vi "Live.Load OPC Tree.vi"(8 "error in (no error)":errorcluster, 9 "Connection.Properties":T1={"Server IP Address"="localhost", "Server Port"=49350, "Message Mode"=enum."None", "Security"=enum."Basic256", "User Name"="", "Password"="", "Client Certificate"=path "", "Server Certificate"=path ""}, 10 "Tree":refnum<vi>, 11 "VI in":refnum<vi>) -> (0 "error out":errorcluster, 3 "LUT":variant)   [LabVIEW 2013, in "OPC UA Client System Explorer.lvlib"]
uses:
  OPC UA Client System Explorer.lvlib
  Shared/Connection.Properties.ctl
  <vilib>/OPCUA/NI OPC UA Client.lvlib
  Shared/OPC UA Client Shared.lvlib
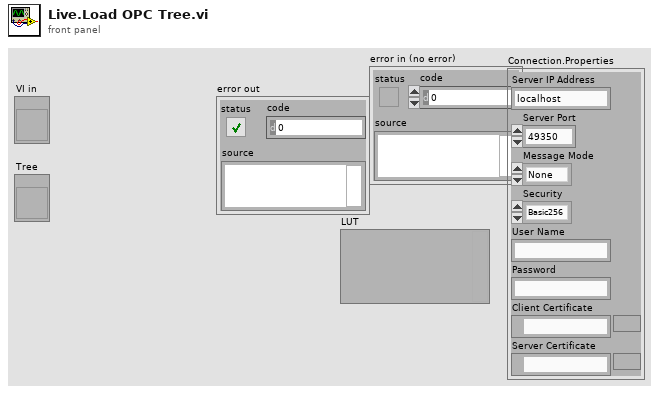
[diagram p1: front panel]
types:
  T1 = typedef "OPC UA Client Shared.lvlib/Connection.Properties.ctl" = cluster{"Server IP Address":string, "Server Port":u16, "Message Mode":enum16{"None", "Sign", "Sign and Encrypt"}, "Security":enum16{"Basic256", "Basic128Rsa15"}, "User Name":string, "Password":string, "Client Certificate":path, "Server Certificate":path}
  T2 = cluster{"message mode":enum16{"None", "Sign", "Sign and Encrypt"}, "security":enum16{"Basic256", "Basic128Rsa15"}}
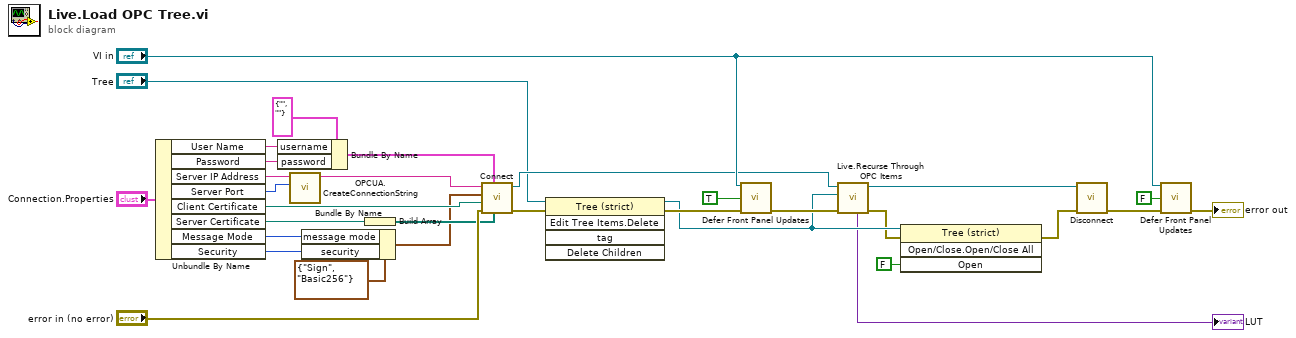
[diagram p0: block diagram]
diagram:
  n1 = Unbundle By Name("Connection.Properties") -> ("User Name"=w11:string, "Password"=w12:string, "Server IP Address"=w15:string, "Server Port"=w14:u16, "Client Certificate"=w8:path, "Server Certificate"=w7:path, "Message Mode"=w3:enum16{"None", "Sign", "Sign and Encrypt"}, "Security"=w2:enum16{"Basic256", "Basic128Rsa15"})
  n2 = Bundle By Name(cluster=cluster{"username":string, "password":string} {"username"="", "password"=""} ("username/password"), "username"=w11, "password"=w12) -> (w9:cluster{"username":string, "password":string})
  n3 = call "OPCUA.CreateConnectionString.vi"("Server Port"=w14, "Server IP Address"=w15) -> ("concatenated string"=w13:string)  [unwired: 9 in]
  n4 = Bundle By Name(cluster=T2 {"message mode"=enum."Sign", "security"=enum."Basic256"} ("security policy"), "message mode"=w3, "security"=w2) -> (w4:T2)
  n5 = Build Array(w7) -> (w6:path[])
  n6 = call <vilib>:"Connect.vi"("trusted server certificates"=w6, "username/password"=w9, "error in (no error)"="error in (no error)", "client certificate file"=w8, "security policy"=w4, "server endpoint URL"=w13) -> ("error out"=w19:errorcluster, "OPC UA client refnum out"=w20:refnum<k21>)  [unwired: 3 in, 1 out]
  n7 = invoke class="Tree (strict)" method="Edit Tree Items.Delete"(reference="Tree", error in=w19) -> (reference out=w25:refnum<vi>, error out=w31:errorcluster)  [unwired: 3 in, 3 out]
  n8 = call "Defer Front Panel Updates.vi"("This VI"="VI in", "Defer Panel Updates"=TRUE, "error in (no error)"=w31) -> ("error out"=w32:errorcluster)  [unwired: 12 in]
  n9 = call "Live.Recurse Through OPC Items.vi"("error in (no error)"=w32, "reference out"=w25, "OPC UA Client Ref"=w20) -> ("error out"=w23:errorcluster, "OPC UA Client Ref"=w21:refnum<k21>, "LUT"=→"LUT":variant)  [unwired: 6 in]
  n10 = invoke class="Tree (strict)" method="Open/Close.Open/Close All"(reference=w25, error in=w23, "Open"=FALSE ("Open?")) -> (error out=w24:errorcluster)  [unwired: 1 in, 3 out]
  n11 = call <vilib>:"Disconnect.vi"("error in (no error)"=w24, "OPC UA client refnum in"=w21) -> ("error out"=w28:errorcluster)  [unwired: 9 in]
  n12 = call "Defer Front Panel Updates.vi"("This VI"="VI in", "Defer Panel Updates"=FALSE, "error in (no error)"=w28) -> ("error out"=→"error out":errorcluster)  [unwired: 12 in]
